vi "File To Line Stream.vi"(11 "file path":path) -> (3 "lines":T1)   [LabVIEW 2023]
uses:
  <extravilib>/ChannelInstances/Stream-str/)Channel.ctl
  <extravilib>/ChannelInstances/Stream-str/Write With Abort.vi
  <extravilib>/ChannelInstances/Stream-str/Endpoint.vi
  <extravilib>/ChannelInstances/Stream-str/)Channel.vi
  <resource>/ChannelSupport/_ChannelSupport/WaitIfNeeded.vi
  <extravilib>/ChannelInstances/Stream-str.lvlib
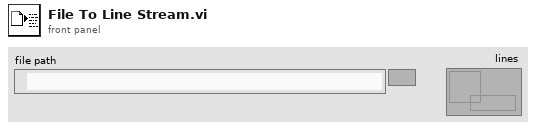
[diagram p1: front panel]
types:
  T1 = typedef "Stream-str.lvlib/)Channel.ctl" = refnum<queue>
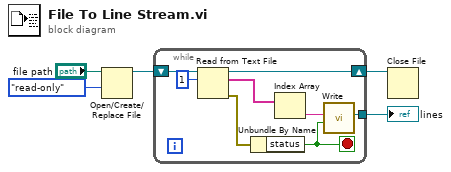
[diagram p0: block diagram]
diagram:
  n1 = Open/Create/Replace File(file path (use dialog)="file path", access (0:read/write)=enum16{"read/write", "read-only", "write-only"}."read-only") -> (refnum out=w3:refnum<file>)  [unwired: 4 in, 2 out]
  n2 = while {
    shift-right: [w13] -> w5
    shift-left: w3 -> [w10]
    tunnel: [w7] -> w2
    stop <- w6 stop-if-true
    n3 = Read from Text File(file (use dialog)=w10, count=1) -> (refnum out=w13:refnum<file>, text=w11:string[], error out=w9:errorcluster)  [unwired: 2 in, 1 out]
    n4 = Unbundle By Name(w9) -> ("status"=w6:bool)
    n5 = Index Array(array=w11) -> (element=w8:string)  [unwired: 1 in]
    n6 = call <extravilib>:"Write.vi"("last element? (F)"=w6, "element"=w8) -> ("channel"=w7:T1)  [unwired: 7 in, 2 out]
  }
  "lines" <- w2
  n7 = Close File(refnum=w5) -> ()  [unwired: 1 in, 2 out]
